vi "Determine PassFail.vi"(0 "Hysteresis Results in":T4[](array[typedef]), 1 "Max Hysteresis %FS":dbl, 2 "Accuracy Results in":T3[](array[typedef]), 3 "Max Accuracy %FS":dbl, 4 "Repeatability Results in":T2[](array[typedef]), 5 "Max Repeatability %FS":dbl, 6 "Linearity Results in":T1[](array[typedef]), 7 "Max Linearity %FS":dbl, 9 "error in (no error)":errorcluster) -> (19 "error out":errorcluster, 20 "Hysteresis Results out":T4[](array[typedef]), 21 "Accuracy Results out":T3[](array[typedef]), 22 "Repeatability Results out":T2[](array[typedef]), 23 "Linearity Results out":T1[](array[typedef]), 24 "Overall PassFail":bool)   [LabVIEW 2026, in "Analysis.lvlib"]
uses:
  Analysis.lvlib
  Hysteresis Result.ctl
  Accuracy Result.ctl
  Repeatability Result.ctl
  Linearity Result.ctl
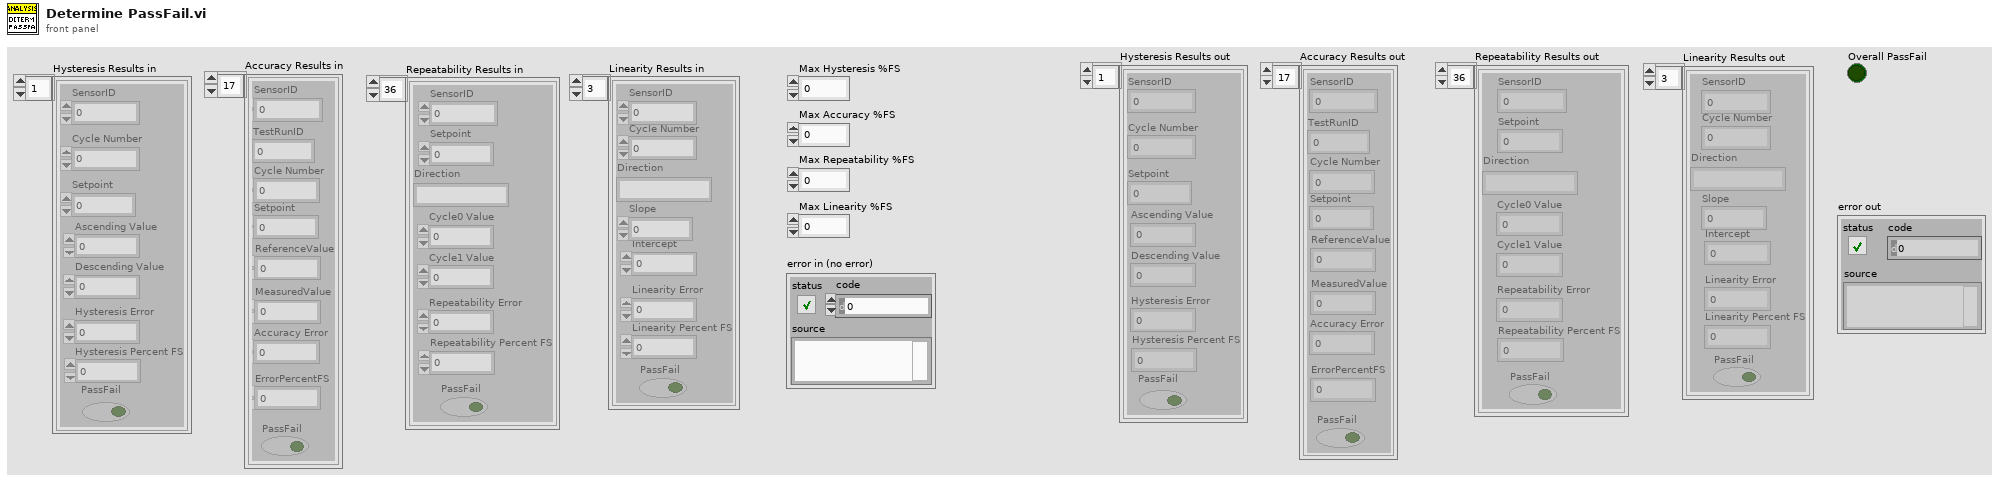
[diagram p1: front panel]
types:
  T1 = typedef "Analysis.lvlib/Linearity Result.ctl" = cluster{"Slope":dbl, "Intercept":dbl, "Cycle Number":i32, "SensorID":i32, "Linearity Error":dbl, "Linearity Percent FS":dbl, "Direction":string, "PassFail":bool}
  T2 = typedef "Analysis.lvlib/Repeatability Result.ctl" = cluster{"Setpoint":dbl, "Cycle0 Value":dbl, "SensorID":i32, "Cycle1 Value":dbl, "Repeatability Error":dbl, "Direction":string, "Repeatability Percent FS":dbl, "PassFail":bool}
  T3 = typedef "Analysis.lvlib/Accuracy Result.ctl" = cluster{"Setpoint":dbl, "Cycle Number":i32, "SensorID":i32, "TestRunID":i32, "ReferenceValue":dbl, "MeasuredValue":dbl, "ErrorPercentFS":dbl, "PassFail":bool, "Accuracy Error":dbl}
  T4 = typedef "Analysis.lvlib/Hysteresis Result.ctl" = cluster{"Setpoint":dbl, "Ascending Value":dbl, "Cycle Number":i32, "SensorID":i32, "Descending Value":dbl, "Hysteresis Error":dbl, "Hysteresis Percent FS":dbl, "PassFail":bool}
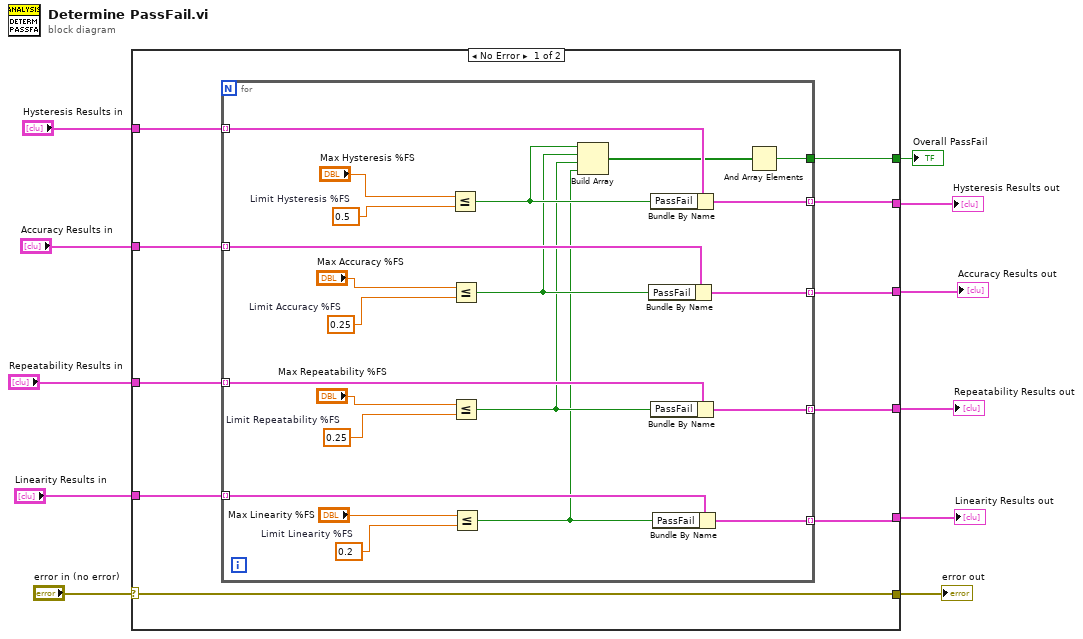
[diagram p0: block diagram]
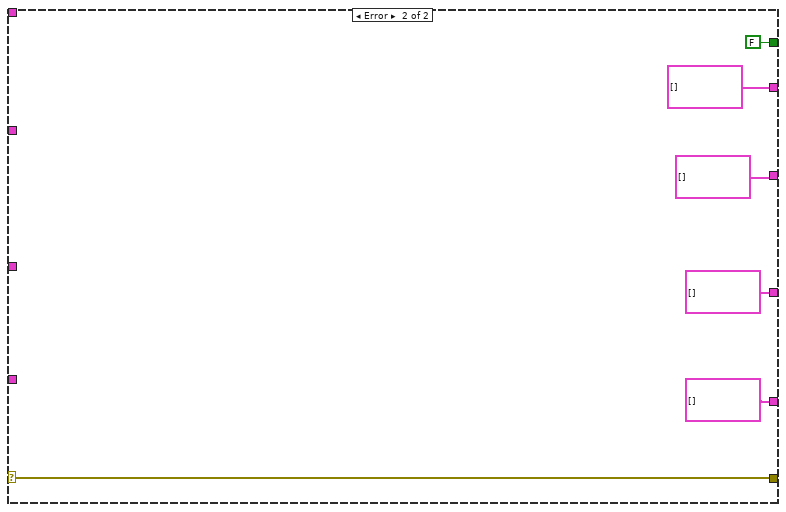
[diagram p2: hidden frame]
diagram:
  n1 = case shown="No Error" "error in (no error)" {
    selector: "error in (no error)" -> [w21 w49]
    tunnel: [w21 w49] -> w10
    tunnel: [w19 T4[] []] -> w9
    tunnel: [w18 T3[] []] -> w8
    tunnel: [w17 T2[] []] -> w7
    tunnel: [w16 T1[] []] -> w6
    tunnel: "Hysteresis Results in" -> [w20 _]
    tunnel: "Accuracy Results in" -> [w15 _]
    tunnel: "Repeatability Results in" -> [w14 _]
    tunnel: "Linearity Results in" -> [w13 _]
    tunnel: [w12 FALSE] -> w1
    frame No Error {
      n2 = for {
        tunnel: w20 -> [w35] mode=indexing
        tunnel: [w34] -> w19 mode=indexing
        tunnel: [w33] -> w18 mode=indexing
        tunnel: [w32] -> w17 mode=indexing
        tunnel: [w31] -> w16 mode=indexing
        tunnel: w15 -> [w30] mode=indexing
        tunnel: w14 -> [w29] mode=indexing
        tunnel: w13 -> [w28] mode=indexing
        tunnel: [w22] -> w12
        w36 = 0.2  # Limit Linearity %FS
        w38 = 0.25  # Limit Repeatability %FS
        w40 = 0.25  # Limit Accuracy %FS
        w42 = 0.5  # Limit Hysteresis %FS
        n3 = Less Or Equal?(x="Max Hysteresis %FS", y=w42) -> (x <= y?=w27:bool)
        n4 = Less Or Equal?(x="Max Accuracy %FS", y=w40) -> (x <= y?=w26:bool)
        n5 = Less Or Equal?(x="Max Repeatability %FS", y=w38) -> (x <= y?=w25:bool)
        n6 = Less Or Equal?(x="Max Linearity %FS", y=w36) -> (x <= y?=w24:bool)
        n7 = Build Array(w27, w26, w25, w24) -> (w23:bool[])
        n8 = Bundle By Name(cluster=w30, "PassFail"=w26) -> (w33:T3)
        n9 = Bundle By Name(cluster=w35, "PassFail"=w27) -> (w34:T4)
        n10 = Bundle By Name(cluster=w29, "PassFail"=w25) -> (w32:T2)
        n11 = Bundle By Name(cluster=w28, "PassFail"=w24) -> (w31:T1)
        n12 = And Array Elements(Boolean array=w23) -> (logical AND=w22:bool)
      }
    }
    frame Error {
    }
  }
  "error out" <- w10
  "Hysteresis Results out" <- w9
  "Accuracy Results out" <- w8
  "Linearity Results out" <- w6
  "Repeatability Results out" <- w7
  "Overall PassFail" <- w1
